vi "LWXPS_PositionerEncoderCalibrationParametersGet.vi"(0 "XPS Reference IN":refnum<k24>, 2 "Positioner Name":string, 5 "LabVIEW error IN":errorcluster) -> (12 "XPS Reference OUT":refnum<k24>, 13 "LabVIEW error OUT":errorcluster, 14 "Returned error code":i32, 15 "Sinus offset":dbl, 16 "Cosinus offset":dbl, 17 "Differential gain":dbl, 18 "Phase compensation":dbl, 19 "XPS Error String":string)   [LabVIEW 2014]
uses:
  D:/XPSQ8_LabView_Library/Development/Source/Dll/Newport.XPS.CommandInterface.dll
  Dll/Newport.XPS.CommandInterface.dll
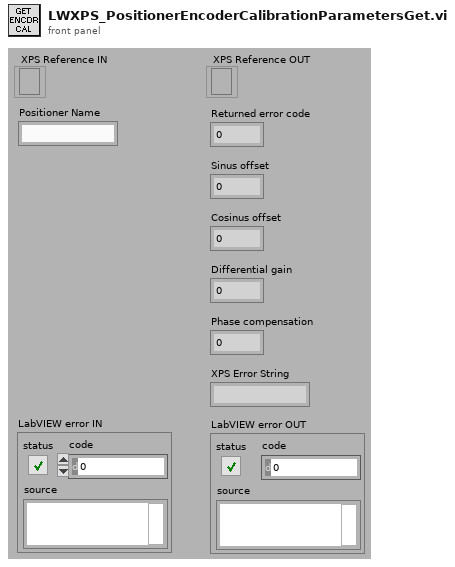
[diagram p1: front panel]
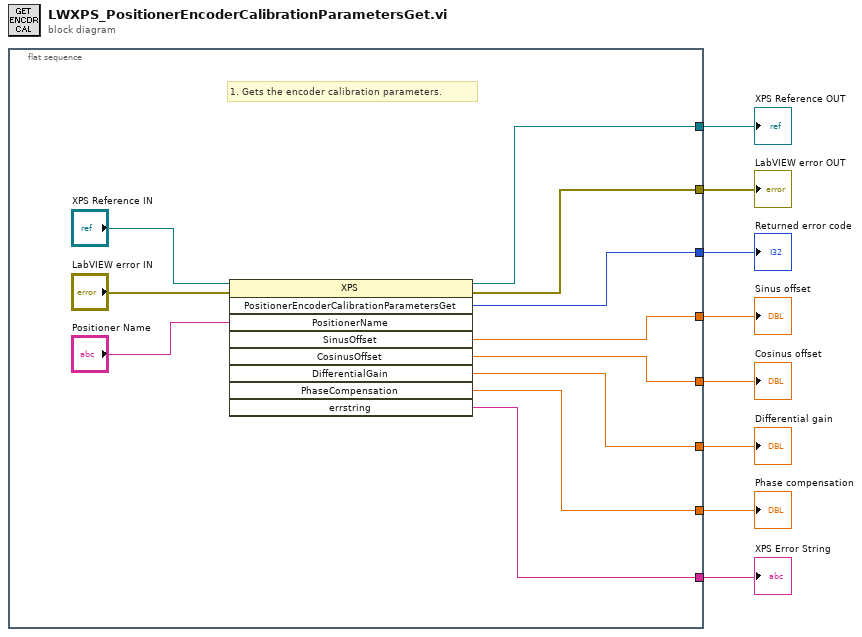
[diagram p0: block diagram]
diagram:
  n1 = flat-sequence {
    tunnel: [w17] -> w8
    tunnel: [w14] -> w7
    tunnel: [w18] -> w6
    tunnel: [w9] -> w1
    tunnel: [w13] -> w5
    tunnel: [w12] -> w4
    tunnel: [w11] -> w2
    tunnel: [w10] -> w3
    frame #0 {
      # "1. Gets the encoder calibration parameters."
      n2 = invoke class="XPS" method="PositionerEncoderCalibrationParametersGet"(reference="XPS Reference IN", error in="LabVIEW error IN", "PositionerName"="Positioner Name") -> (reference out=w17:refnum<k24>, error out=w14:errorcluster, "PositionerEncoderCalibrationParametersGet"=w18:i32, "SinusOffset"=w9:dbl, "CosinusOffset"=w13:dbl, "DifferentialGain"=w12:dbl, "PhaseCompensation"=w11:dbl, "errstring"=w10:string)  [unwired: 6 in, 1 out]
    }
  }
  "XPS Error String" <- w3
  "XPS Reference OUT" <- w8
  "LabVIEW error OUT" <- w7
  "Returned error code" <- w6
  "Cosinus offset" <- w5
  "Differential gain" <- w4
  "Phase compensation" <- w2
  "Sinus offset" <- w1
